vi "receiver.vi"() -> ()   [LabVIEW 2026]
uses:
  <instrlib>/niUSRP/niUSRP Fetch Rx Data (CDB Cluster).vi
  <vilib>/addons/Modulation/niAMT.lvlib
panel:
  out "Imaginary Part":waveform(dbl)(graph)
  out "Real Part":waveform(dbl)(graph)
  in  "stop":bool
  in  "number of samples":i64
  out "coerced gain":dbl format="%#_6f"
  out "coerced carrier frequency":dbl=100000.0 format="%#_6p"
  out "coerced IQ rate":dbl=100000.0 format="%#_6p"
  in  "active antenna":string
  in  "gain":dbl format="%#_6f"
  in  "carrier frequency":dbl=100000.0 format="%#_6p"
  in  "IQ rate":dbl=100000.0 format="%#_6p"
  in  "IP ADDRESS":refnum<k15>
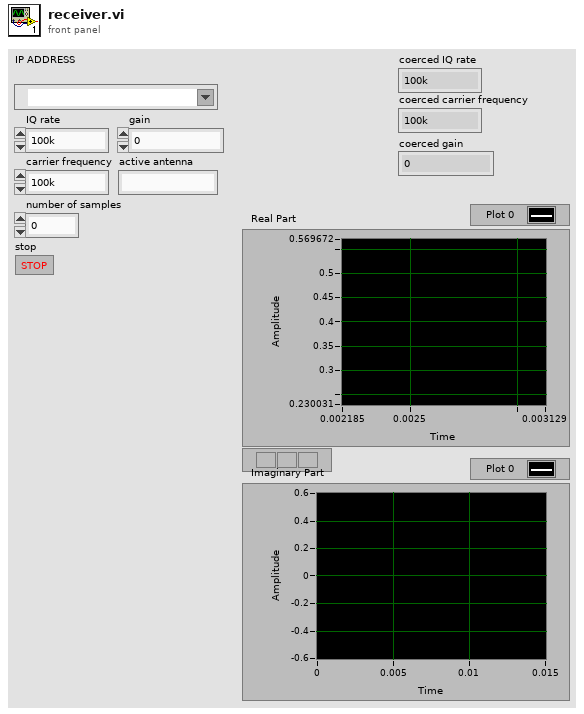
[diagram p1: front panel]
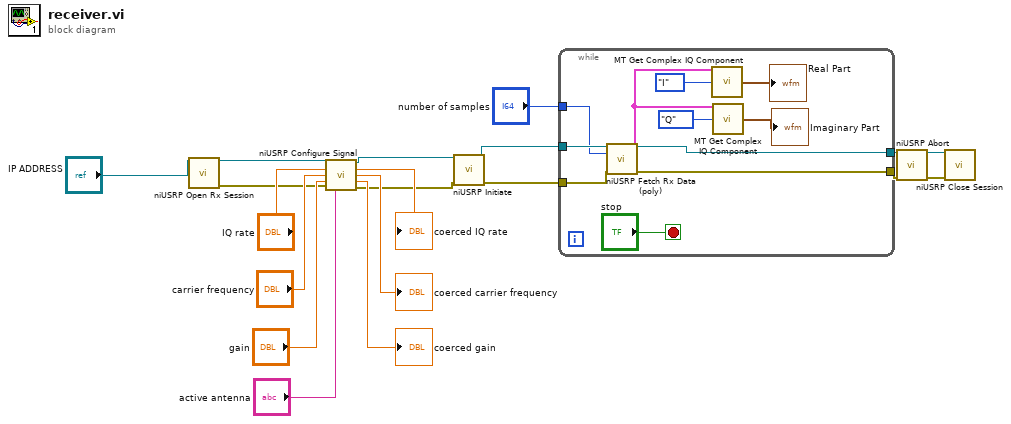
[diagram p0: block diagram]
diagram:
  n1 = call <instrlib>:"niUSRP Open Rx Session.vi"("device names"="IP ADDRESS") -> ("session handle out"=w2:refnum<k15>, "error out"=w11:errorcluster)  [unwired: 13 in]
  n2 = call <instrlib>:"niUSRP Configure Signal.vi"("session handle"=w2, "IQ rate"="IQ rate", "carrier frequency"="carrier frequency", "gain"="gain", "error in (no error)"=w11, "active antenna"="active antenna") -> ("session handle out"=w3:refnum<k15>, "coerced IQ rate"=→"coerced IQ rate":dbl, "coerced carrier frequency"=→"coerced carrier frequency":dbl, "coerced gain"=→"coerced gain":dbl, "error out"=w10:errorcluster)  [unwired: 5 in]
  n3 = call <instrlib>:"niUSRP Initiate.vi"("session handle"=w3, "error in (no error)"=w10) -> ("session handle out"=w4:refnum<k15>, "error out"=w9:errorcluster)  [unwired: 12 in]
  n4 = while {
    tunnel: w9 -> [w30]
    tunnel: [w29] -> w8
    tunnel: [w28] -> w5
    tunnel: w4 -> [w27]
    tunnel: "number of samples" -> [w26]
    stop <- "stop" stop-if-true
    n5 = call-poly <instrlib>:"niUSRP Fetch Rx Data (poly).vi"("session handle"=w27, "number of samples"=w26, "error in (no error)"=w30) -> ("session handle out"=w28:refnum<k15>, "data"=w21:cluster{"t0":dbl, "dt":dbl, "Y":cdb[]}, "error out"=w29:errorcluster)  [unwired: 9 in, 1 out]
    n6 = call <vilib>:"MT Get Complex IQ Component.vi"("IQ data (complex) in"=w21, "component choice"=enum16{"I", "Q", "Magnitude", "Phase"}."I") -> ("CE component"=→"Real Part":waveform(dbl))  [unwired: 11 in, 2 out]
    n7 = call <vilib>:"MT Get Complex IQ Component.vi"("IQ data (complex) in"=w21, "component choice"=enum16{"I", "Q", "Magnitude", "Phase"}."Q") -> ("CE component"=→"Imaginary Part":waveform(dbl))  [unwired: 11 in, 2 out]
  }
  n8 = call <instrlib>:"niUSRP Abort.vi"("session handle"=w5, "error in (no error)"=w8) -> ("session handle out"=w6:refnum<k15>, "error out"=w7:errorcluster)  [unwired: 12 in]
  n9 = call <instrlib>:"niUSRP Close Session.vi"("session handle"=w6, "error in (no error)"=w7) -> ()  [unwired: 13 in, 1 out]
